vi "Add Axes.vi"(11 "robot elements in":T1[](array[typedef])) -> (3 "robot elements out":T1[](array[typedef]))   [LabVIEW 2017, in "NI_Kinematics.lvlib"]
uses:
  <vilib>/robotics/Kinematics/NI_Kinematics.lvlib
  <vilib>/robotics/Kinematics/Plotting/Tree Element.ctl
  <vilib>/robotics/Kinematics/Plotting/Element Type.ctl
  <vilib>/robotics/Kinematics/Plotting/Joint Type.ctl
  <vilib>/robotics/Kinematics/Plotting/NI_Robotics_3DKinematics.lvlib
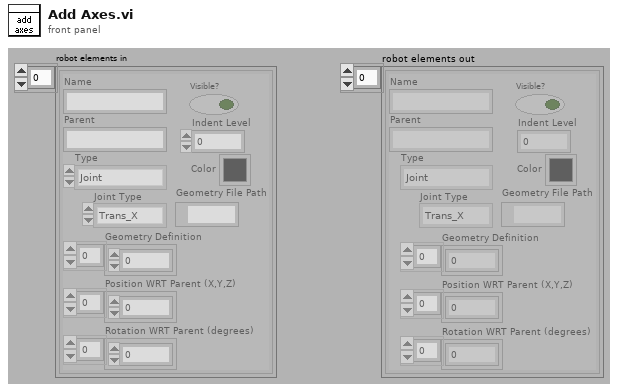
[diagram p1: front panel]
types:
  T1 = typedef "NI_Robotics_3DKinematics.lvlib/Tree Element.ctl" = cluster{"Name":string, "Parent":string, "Type":T2, "Visible?":bool, "Geometry Definition":dbl[], "Position WRT Parent (X,Y,Z)":dbl[], "Rotation WRT Parent (degrees)":dbl[], "Joint Type":T3, "Geometry File Path":path, "Indent Level":i32, "Color":u32}
  T2 = typedef "NI_Robotics_3DKinematics.lvlib/Element Type.ctl" = enum16{"Joint", "Box", "Cylinder", "Cone", "Sphere", "ASE File", "VRML File", "STL File", "Space"}
  T3 = typedef "NI_Robotics_3DKinematics.lvlib/Joint Type.ctl" = enum16{"Trans_X", "Trans_Y", "Trans_Z", "Rot_X", "Rot_Y", "Rot_Z", "None"}
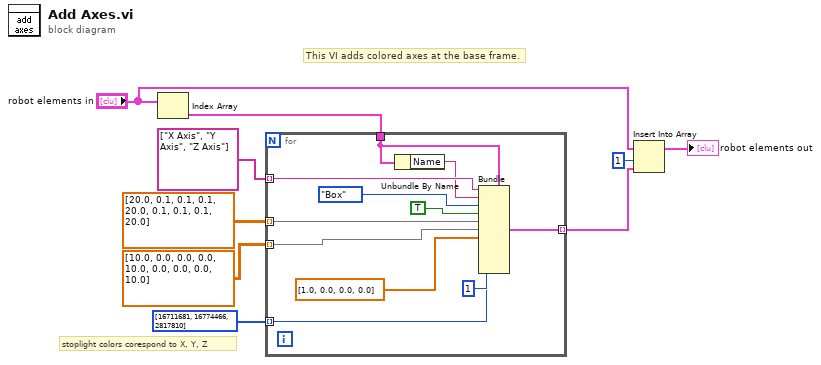
[diagram p0: block diagram]
diagram:
  # "stoplight colors corespond to X, Y, Z"
  # "This VI adds colored axes at the base frame."
  n1 = Index Array(array="robot elements in") -> (element=w3:T1)  [unwired: 1 in]
  n2 = for {
    tunnel: dbl[][] [[20.0, 0.1, 0.1], [0.1, 20.0, 0.1], [0.1, 0.1, 20.0]] ("Rotation WRT Parent (degrees)") -> [w16] mode=indexing
    tunnel: string[] ["X Axis", "Y Axis", "Z Axis"] ("Rotation WRT Parent (degrees)") -> [w15] mode=indexing
    tunnel: [w14] -> w6 mode=indexing
    tunnel: w3 -> [w12]
    tunnel: u32[] [16711681, 16774466, 2817810] ("Rotation WRT Parent (degrees)") -> [w11] mode=indexing
    tunnel: dbl[][] [[10.0, 0.0, 0.0], [0.0, 10.0, 0.0], [0.0, 0.0, 10.0]] ("Rotation WRT Parent (degrees)") -> [w10] mode=indexing
    n3 = Unbundle By Name(w12) -> ("Name"=w13:string)
    n4 = Bundle(cluster=w12, "Name"=w15, "Parent"=w13, "Type"=Element_Type."Box", "Visible?"=TRUE ("Visable?"), "Geometry Definition"=w16, "Position WRT Parent (X,Y,Z)"=w10, "Rotation WRT Parent (degrees)"=dbl[] [1.0, 0.0, 0.0, 0.0], "Indent Level"=1, "Color"=w11) -> (w14:T1)  [unwired: 2 in]
  }
  n5 = Insert Into Array(array="robot elements in", index=1, new element=w6) -> (→"robot elements out":T1[])
